vi "Set Measurement Name.vi"(8 "error in (no error)":errorcluster, 11 "QPA Measurement in":refnum<class "QPA Measurement.lvclass">) -> (0 "error out":errorcluster, 3 "QPA Measurement out":refnum<class "QPA Measurement.lvclass">)   [LabVIEW 2016, in "QPA Measurement.lvlib" / "QPA Measurement.lvclass"]
uses:
  QPA Measurement.lvclass
  C:/Projects/STS/Common/Sequence Automation/Plugins/Measurement Interface.lvlibp/Measurement Interface.lvclass
  QPA Measurement.lvclass/QPA Measurement.ctl
  Plugins/Measurement Interface.lvlibp/Private Methods/Measurement Parameters/Read Measurement Parameters.vi
  Plugins/String Database.lvlibp/String Database.lvclass
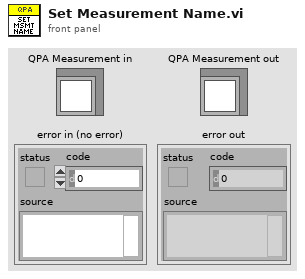
[diagram p1: front panel]
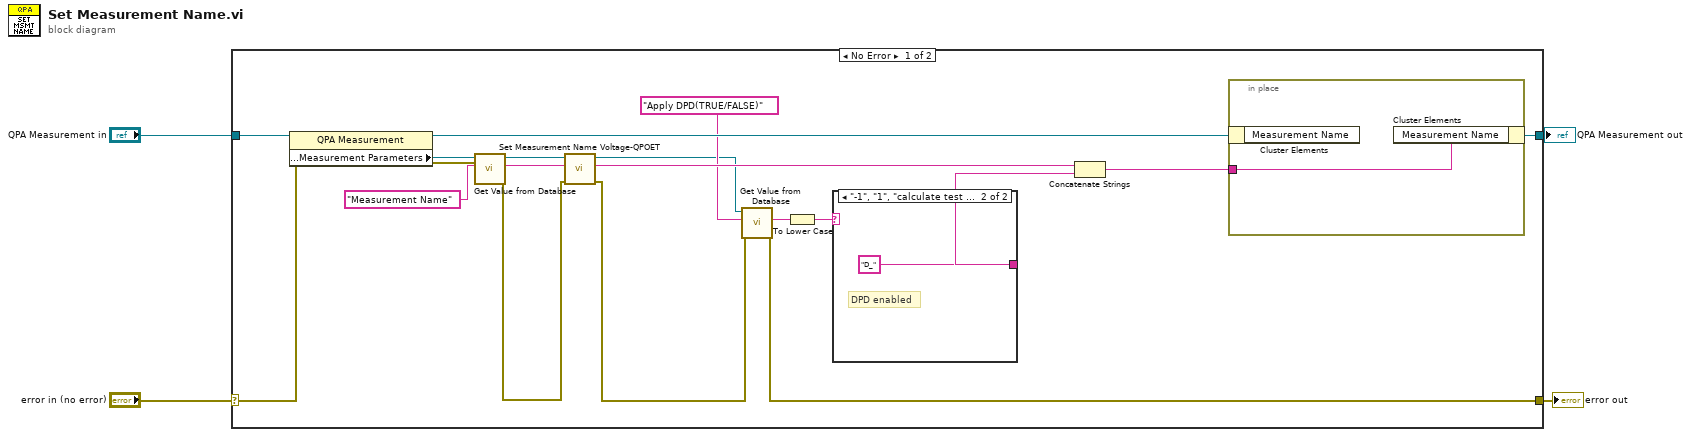
[diagram p0: block diagram]
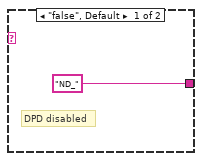
[diagram p2: hidden frame]
diagram:
  n1 = case shown="No Error" "error in (no error)" {
    selector: "error in (no error)" -> [w23 w28]
    tunnel: [w6 w28] -> w3
    tunnel: [w16 w27] -> w1
    tunnel: "QPA Measurement in" -> [w22 w27]
    frame No Error {
      n2 = property class="QPA Measurement"(reference=w22, error in=w23) -> (reference out=w17:refnum<class "QPA Measurement.lvclass">, error out=w20:errorcluster, "Protected Methods:Measurement Parameters"=w21:refnum<class "String Database.lvclass">)
      n3 = call "Get Value from Database.vi"("error in (no error)"=w20, "Entry Name"="Measurement Name", "Message in"=w21) -> ("error out"=w19:errorcluster, "Entry Value"=w13:string, "Message out"=w14:refnum<class "String Database.lvclass">)  [unwired: 5 in, 1 out]
      n4 = call "Set Measurement Name Voltage-QPOET.vi"("error in (no error)"=w19, "Meas Name In"=w13, "Message in"=w14) -> ("error out"=w7:errorcluster, "Meas Name Out"=w15:string, "Message out"=w10:refnum<class "String Database.lvclass">)  [unwired: 6 in]
      n5 = call "Get Value from Database.vi"("error in (no error)"=w7, "Entry Name"="Apply DPD(TRUE/FALSE)", "Message in"=w10) -> ("error out"=w6:errorcluster, "Entry Value"=w11:string)  [unwired: 5 in, 2 out]
      n6 = To Lower Case(string=w11) -> (all lower case string=w5:string)
      n7 = case shown="\"-1\", \"1\", \"calculate test group lut\", \"true\", \"use test group lut\"" w5 {
        tunnel: ["ND_" ("Entry Value") "D_" ("Entry Value")] -> w8
        frame "false", Default {
          # "DPD disabled"
        }
        frame "-1", "1", "calculate test group lut", "true", "use test group lut" {
          # "DPD enabled"
        }
      }
      n8 = Concatenate Strings(w15, w8) -> (w9:string)
      n9 = in-place {
        in-place-border: w9 -> [w26]
        n10 = in-place-cluster #1(w17) -> ()  [unwired: 1 out]
        n11 = in-place-cluster #1("Measurement Name"=w26) -> (w16:refnum<class "QPA Measurement.lvclass">)
      }
    }
    frame Error {
    }
  }
  "error out" <- w3
  "QPA Measurement out" <- w1
